vi "Create_setup_string.vi"() -> (0 "Setup String":string)   [LabVIEW 2017]
uses:
  Globals/Meas_global.vi
  Globals/Trav_pos_global.vi
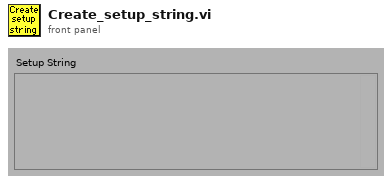
[diagram p1: front panel]
types:
  T1 = typedef "Analysis_info_cluster.ctl" = cluster{"Colour":u32, "Inst type":T2, "Inst name":string, "Symbol":string, "Code name":string, "Extra Info":string, "Inst Array":T3, "Extra Titles":string[], "Extra Values":string[], "U":dbl, "u^2":dbl, "u^3":dbl, "u^4":dbl, "Skew_u":dbl, "Kurt_u":dbl, "Sd Error in Mean":dbl, "% u'/U":dbl, "X":dbl, "Y":dbl, "Z":dbl, "Timescale integral Estimate":dbl, "Sd Error in Variance":dbl, "Calib File":path, "Calib Constants":dbl[], "Output Position":bool, "Full Stats":bool, "Av Sampling Rate":dbl, "Av No of Samples":dbl, "Total Meas Time (s)":dbl, "ADAM Ch Name":string, "Max value":dbl, "Min value":dbl, "Req Sample Rate Hz":dbl, "Sync Delay Time (s)":dbl, "Ch No":i16, "Device ID":string, "Use Latest Calib":bool}
  T2 = typedef "Inst_type.ctl" = enum16{"Propeller anemometer", "Raw voltage", "Pressure Transducer", "Pitot-static tube", "Preston tube", "Hot wire", "Cross wire 1", "Cross wire 2", "Generic Linear", "Generic Polynomial", "Generic BackPoly", "Fast FID", "Thermocouple", "Cold wire", "Pulsed Wire", "LDA Vel", "LDA Tran time", "LDA Arr time", "Microphone"}
  T3 = typedef "Instrument_Array.ctl" = enum16{"PWA", "LDA", "Analogue"}
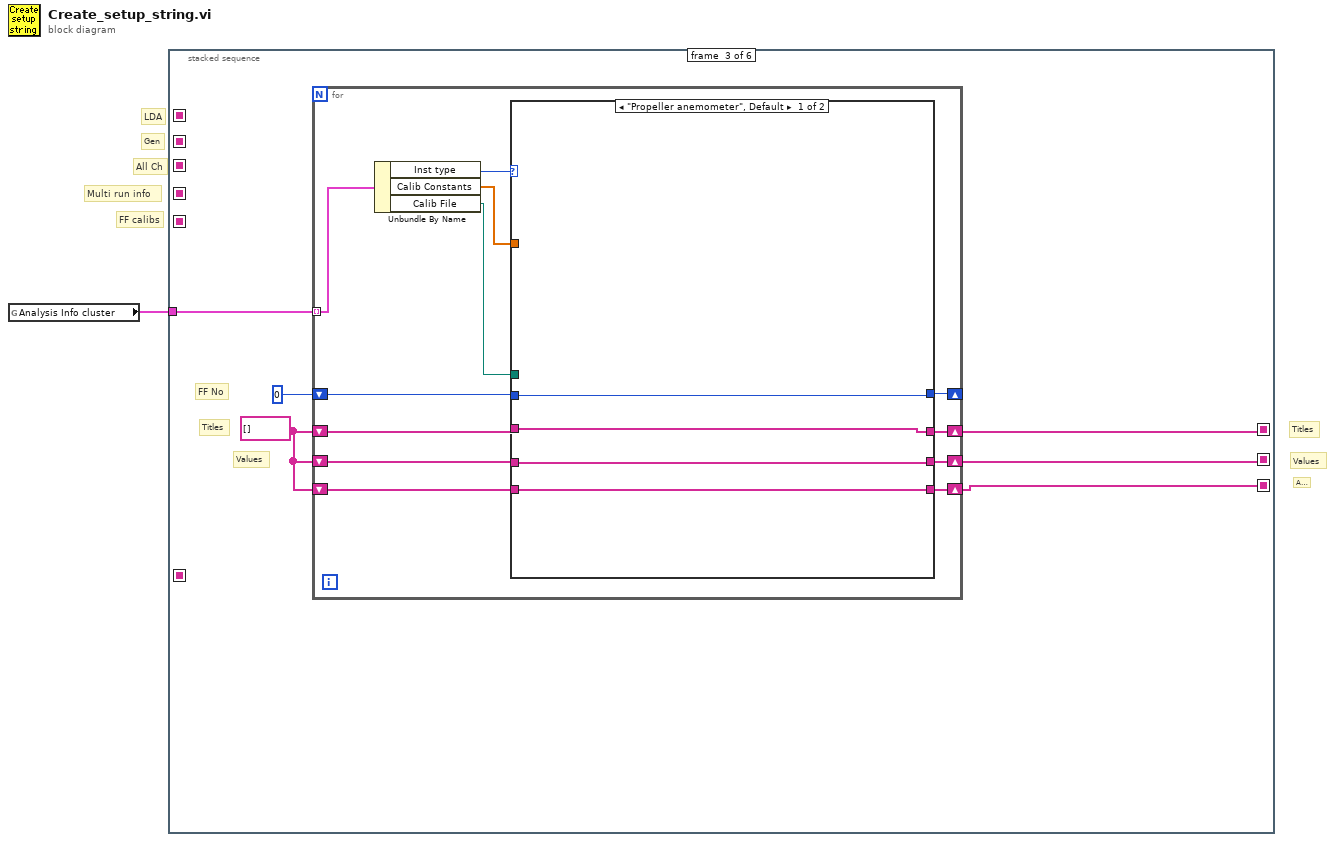
[diagram p0: block diagram]
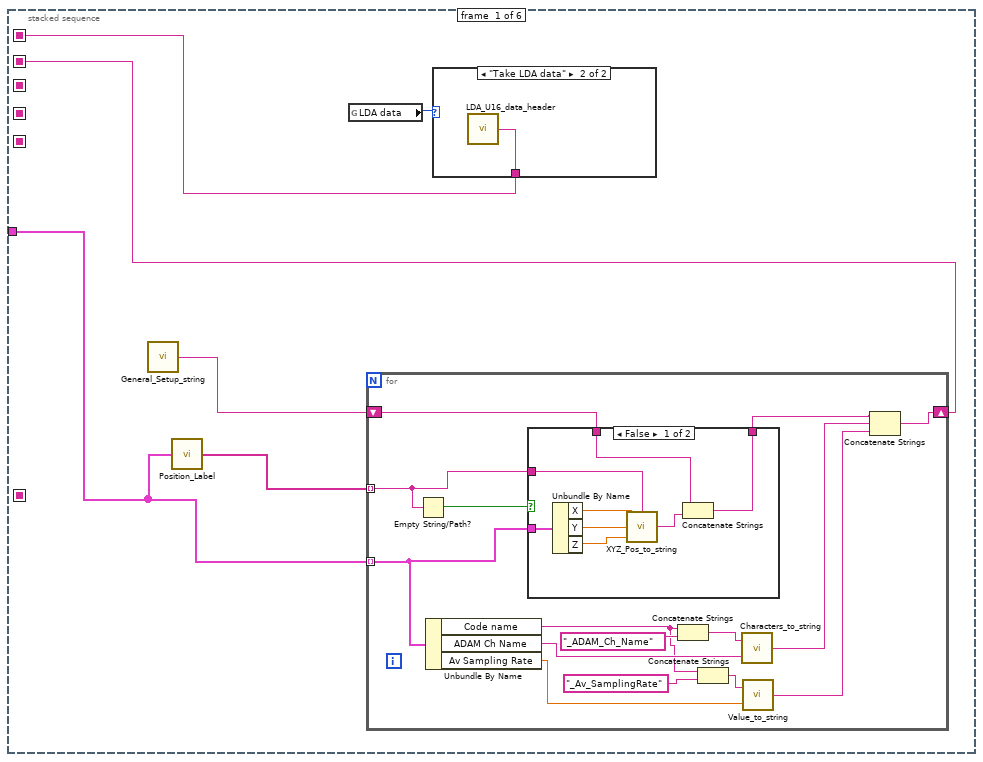
[diagram p2: hidden frame]
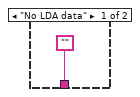
[diagram p4: hidden frame]
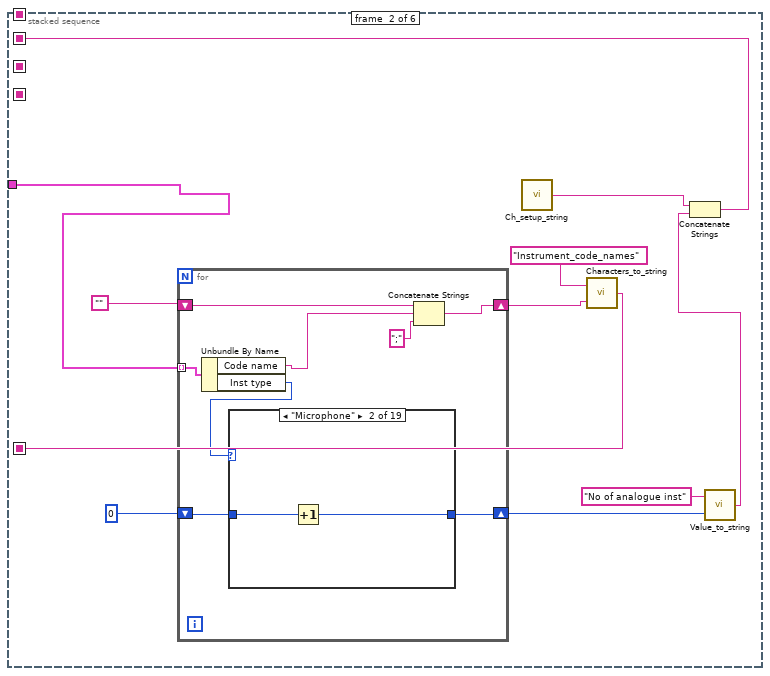
[diagram p5: hidden frame]
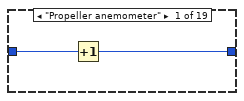
[diagram p6: hidden frame]
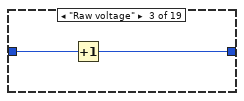
[diagram p7: hidden frame]
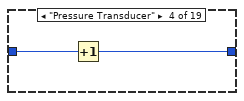
[diagram p8: hidden frame]
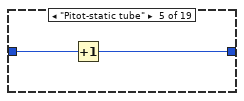
[diagram p9: hidden frame]
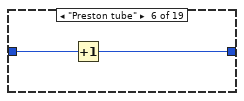
[diagram p10: hidden frame]
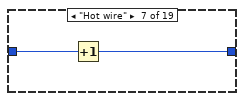
[diagram p11: hidden frame]
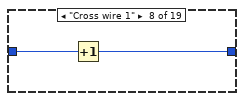
[diagram p12: hidden frame]
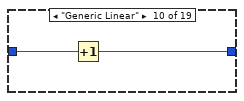
[diagram p14: hidden frame]
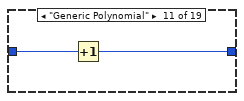
[diagram p15: hidden frame]
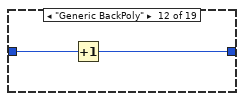
[diagram p16: hidden frame]
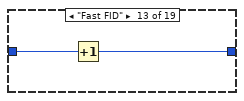
[diagram p17: hidden frame]
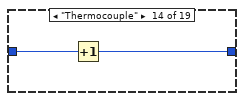
[diagram p18: hidden frame]
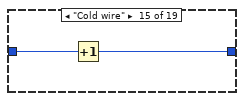
[diagram p19: hidden frame]
diagram:
  # "Multi run info"
  # "After"
  # "Values"
  # "Titles"
  # "FF calibs"
  # "LDA"
  # "Gen"
  # "All Ch"
  n1 = global read "Meas_global.vi" "Analysis Info cluster"() -> (w1:T1[])
  n2 = stacked-sequence {
    seq-local: [w7 _ _ _ _ _] -> [_ _ _ _ _ w221]
    seq-local: [w3 _ _ _ _ _] -> [_ _ _ _ _ w220]
    seq-local: [_ w35 _ _ _ _] -> [_ _ _ _ _ w219]
    seq-local: [_ _ _ _ w167 _] -> [_ _ _ _ _ w194]
    seq-local: [_ _ w89 _ _ _] -> [_ _ _ _ w168 _]
    seq-local: [_ _ w90 _ _ _] -> [_ _ _ _ w165 _]
    seq-local: [_ _ w87 _ _ _] -> [_ _ _ _ w163 _]
    seq-local: [_ w41 _ _ _ _] -> [_ _ _ _ _ w200]
    seq-local: [_ _ _ w155 _ _] -> [_ _ _ _ _ w193]
    tunnel: w1 -> [w2 w34 w86 _ _ _]
    frame #0 {
      n3 = call "General_Setup_string.vi"() -> ("Output string"=w4:string)  [unwired: 1 out]
      n4 = call "Position_Label.vi"("Analysis Info cluster"=w2) -> ("Position Label"=w5:string[])
      n5 = global read "Meas_global.vi" "LDA data"() -> (w6:enum16{"No LDA data", "Take LDA data"})
      n6 = for {
        shift-right: [w18] -> w3
        shift-left: w4 -> [w22]
        tunnel: w2 -> [w17] mode=indexing
        tunnel: w5 -> [w21] mode=indexing
        n7 = Empty String/Path?(string/path=w21) -> (empty?=w20:bool)
        n8 = Unbundle By Name(w17) -> ("Code name"=w11:string, "ADAM Ch Name"=w14:string, "Av Sampling Rate"=w12:dbl)
        n9 = case shown="False" w20 {
          tunnel: w22 -> [w30 w31]
          tunnel: [w29 w31] -> w19
          tunnel: w17 -> [w28 _]
          tunnel: w21 -> [w23 _]
          frame False {
            n10 = Unbundle By Name(w28) -> ("X"=w25:dbl, "Y"=w26:dbl, "Z"=w27:dbl)
            n11 = call "XYZ_Pos_to_string.vi"("Position label"=w23, "Z"=w27, "Y"=w26, "X"=w25) -> ("Output string"=w24:string)
            n12 = Concatenate Strings(w30, w24) -> (w29:string)
          }
          frame True {
          }
        }
        n13 = Concatenate Strings(w11, "_ADAM_Ch_Name" ("string")) -> (w15:string)
        n14 = Concatenate Strings(w11, "_Av_SamplingRate" ("string")) -> (w9:string)
        n15 = call "Characters_to_string.vi"("Characters to write"=w14, "Label for characters"=w15) -> ("Output string"=w13:string)
        n16 = call "Value_to_string.vi"("Value"=w12, "Label for value"=w9) -> ("Output string"=w8:string)  [unwired: 1 in]
        n17 = Concatenate Strings(w19, w13, w8) -> (w18:string)
      }
      n18 = case shown="\"Take LDA data\"" w6 {
        tunnel: ["" w33] -> w7
        frame "No LDA data" {
        }
        frame "Take LDA data" {
          n19 = call "LDA_U16_data_header.vi"() -> ("Output string"=w33:string)  [unwired: 1 out]
        }
      }
    }
    frame #1 {
      n20 = for {
        tunnel: w34 -> [w52] mode=indexing
        shift-right: [w48] -> w43
        shift-left: "" -> [w51]
        shift-right: [w45] -> w38
        shift-left: 0 -> [w46]
        n21 = Unbundle By Name(w52) -> ("Code name"=w50:string, "Inst type"=w47:T2)
        n22 = case shown="\"Microphone\"" w47 {
          tunnel: w46 -> [w54 w56 w58 w60 w62 w64 w66 w68 w69 w71 w73 w75 w77 w79 w81 w82 w83 w84 w85]
          tunnel: [w53 w55 w57 w59 w61 w63 w65 w67 w69 w70 w72 w74 w76 w78 w80 w82 w83 w84 w85] -> w45
          frame "Propeller anemometer" {
            n23 = Increment(x=w54) -> (x+1=w53:i32)
          }
          frame "Microphone" {
            n24 = Increment(x=w56) -> (x+1=w55:i32)
          }
          frame "Raw voltage" {
            n25 = Increment(x=w58) -> (x+1=w57:i32)
          }
          frame "Pressure Transducer" {
            n26 = Increment(x=w60) -> (x+1=w59:i32)
          }
          frame "Pitot-static tube" {
            n27 = Increment(x=w62) -> (x+1=w61:i32)
          }
          frame "Preston tube" {
            n28 = Increment(x=w64) -> (x+1=w63:i32)
          }
          frame "Hot wire" {
            n29 = Increment(x=w66) -> (x+1=w65:i32)
          }
          frame "Cross wire 1" {
            n30 = Increment(x=w68) -> (x+1=w67:i32)
          }
          frame "Cross wire 2" {
          }
          frame "Generic Linear" {
            n31 = Increment(x=w71) -> (x+1=w70:i32)
          }
          frame "Generic Polynomial" {
            n32 = Increment(x=w73) -> (x+1=w72:i32)
          }
          frame "Generic BackPoly" {
            n33 = Increment(x=w75) -> (x+1=w74:i32)
          }
          frame "Fast FID" {
            n34 = Increment(x=w77) -> (x+1=w76:i32)
          }
          frame "Thermocouple" {
            n35 = Increment(x=w79) -> (x+1=w78:i32)
          }
          frame "Cold wire" {
            n36 = Increment(x=w81) -> (x+1=w80:i32)
          }
          frame "Pulsed Wire" {
          }
          frame "LDA Vel" {
          }
          frame "LDA Tran time" {
          }
          frame "LDA Arr time" {
          }
        }
        n37 = Concatenate Strings(w51, w50, ";" ("string")) -> (w48:string)
      }
      n38 = call "Ch_setup_string.vi"() -> ("Output string"=w37:string)  [unwired: 3 in, 3 out]
      n39 = call "Characters_to_string.vi"("Characters to write"=w43, "Label for characters"="Instrument_code_names") -> ("Output string"=w41:string)
      n40 = call "Value_to_string.vi"("Value"=w38, "Label for value"="No of analogue inst") -> ("Output string"=w36:string)  [unwired: 1 in]
      n41 = Concatenate Strings(w37, w36) -> (w35:string)
    }
    frame #2 {
      w88 = string[] []
      # "Values"
      # "Titles"
      # "FF No"
      n42 = for {
        shift-right: [w99] -> w89
        shift-left: w88 -> [w100]
        shift-right: [w101] -> _
        shift-left: 0 -> [w102]
        shift-right: [w97] -> w90
        shift-left: w88 -> [w98]
        shift-right: [w95] -> w87
        shift-left: w88 -> [w96]
        tunnel: w86 -> [w92] mode=indexing
        n43 = Unbundle By Name(w92) -> ("Inst type"=w103:T2, "Calib Constants"=w94:dbl[], "Calib File"=w93:path)
        n44 = case shown="\"Propeller anemometer\", Default" w103 {
          tunnel: w94 -> [_ w117]
          tunnel: w93 -> [_ w116]
          tunnel: w102 -> [w107 w115]
          tunnel: [w107 w114] -> w101
          tunnel: w100 -> [w106 w113]
          tunnel: [w106 w112] -> w99
          tunnel: w98 -> [w105 w111]
          tunnel: [w105 w110] -> w97
          tunnel: w96 -> [w104 w109]
          tunnel: [w104 w108] -> w95
          frame "Propeller anemometer", Default {
          }
          frame "Fast FID" {
            n45 = stacked-sequence {
              seq-local: [w118 _] -> [_ w140]
              tunnel: w117 -> [_ w153]
              tunnel: w116 -> [_ w154]
              tunnel: w115 -> [w133 _]
              tunnel: [w118 _] -> w114
              tunnel: w113 -> [w129 _]
              tunnel: [w128 _] -> w112
              tunnel: w111 -> [_ w148]
              tunnel: [_ w147] -> w110
              tunnel: w109 -> [_ w145]
              tunnel: [_ w144] -> w108
              frame #0 {
                # "Titles"
                n46 = Increment(x=w133) -> (x+1=w118:i32)
                n47 = Number To Decimal String(number=w118) -> (decimal integer string=w119:string)  [unwired: 1 out]
                n48 = Build Array("Calib Filename", "Coeff A", "Coeff B", "Coeff C", "Bkgnd", "Bkgnd Variance", "Bkgnd Volts", "Bkgnd Time") -> (w130:string[])
                n49 = for {
                  tunnel: "FF:" -> [w138]
                  tunnel: w119 -> [w137]
                  tunnel: w130 -> [w135] mode=indexing
                  tunnel: [w134] -> w122 mode=indexing
                  n50 = Concatenate Strings(w138, w137, ":" ("Substring"), w135) -> (w134:string)
                }
                n51 = Build Array (concatenate)(w129, w122) -> (w128:string[])
              }
              frame #1 {
                n52 = Array Subset(array=w153, length=7 ("Array Length")) -> (w151:dbl[])  [unwired: 1 in]
                n53 = Initialize Array("", 4 ("dimension size")) -> (w141:string[])
                n54 = call "Bkgnd_place_names.vi"("Numeric"=w140) -> ("Array"=w139:string[])
                n55 = Path To String(path=w154) -> (string=w146:string)
                n56 = Number To Fractional String(number=w151, precision (6)=i16 10) -> (F-format string=w149:string[])  [unwired: 2 out]
                n57 = Build Array (concatenate)(w148, w146, w149) -> (w147:string[])
                n58 = Build Array (concatenate)(w145, w141, w139) -> (w144:string[])
              }
            }
          }
        }
      }
    }
    frame #3 {
      n59 = global read "Trav_pos_global.vi" "Current Image Filename"() -> (w160:path)
      n60 = global read "Meas_global.vi" "Extra command String"() -> (w162:string)
      n61 = call "Path_2_String.vi"("Real Path"=w160) -> ("Path String"=w159:string)
      n62 = call "Characters_to_string.vi"("Characters to write"=w162, "Label for characters"="Meas_Global.vi_Extra Command String") -> ("Output string"=w157:string)
      n63 = call "Characters_to_string.vi"("Characters to write"=w159, "Label for characters"="Trav_pos_global.vi_Current Image Filename") -> ("Output string"=w156:string)
      n64 = Concatenate Strings(w157, w156) -> (w155:string)
    }
    frame #4 {
      n65 = Array Size(array=w165) -> (size(s)=w166:i32)
      n66 = Not Equal To 0?(x=w166) -> (x != 0?=w164:bool)
      n67 = case shown="True" w164 {
        tunnel: w168 -> [_ w185]
        tunnel: w165 -> [_ w179]
        tunnel: ["" w173] -> w167
        tunnel: w163 -> [_ w171]
        frame False {
        }
        frame True {
          n68 = Build Array (concatenate)("FF:Calib:History" ("Input Element"), w185) -> (w176:string[])
          n69 = for {
            tunnel: w176 -> [w192] mode=indexing
            tunnel: [w191] -> w188 mode=indexing
            tunnel: [w190] -> w187 mode=indexing
            tunnel: [w189] -> w186 mode=indexing
            n70 = call "Split_Ch_name.vi"("Ch name"=w192) -> ("Top level"=w191:string, "Middle"=w190:string, "Low level"=w189:string)
          }
          n71 = Build Array (concatenate)("Calibration To be Used" ("Input Element"), w179) -> (w181:string[])
          n72 = call "Asterisk_header.vi"("Channel names"=w176) -> ("Header string"=w174:string)
          n73 = Build Array (concatenate)("Calibration After Meas" ("Input Element"), w171) -> (w170:string[])
          n74 = Build Array (concatenate)("Calibration Before Meas" ("Input Element"), w179) -> (w182:string[])
          n75 = Build Array(w188, w187, w186, w182, w170, w181) -> (w177:string[][])
          n76 = Array To Spreadsheet String(array=w177, 3:"%s" ("format string")) -> (spreadsheet string=w175:string)  [unwired: 1 out]
          n77 = Concatenate Strings(w174, w175) -> (w173:string)
        }
      }
    }
    frame #5 {
      w195 = "Initial Probe positions" ("File Label")
      n78 = global read "Meas_global.vi" "Pre Setup String"() -> (w199:string)
      n79 = Get Date/Time In Seconds() -> (seconds since 1Jan1904=w207:timestamp)
      n80 = To Double Precision Float(number=w207) -> (double precision float=w209:dbl)
      n81 = global read "Meas_global.vi" "New Setup String"() -> (w197:string)
      n82 = global read "Meas_global.vi" "Results file"() -> (w216:path)
      n83 = call "Get_string_subset.vi"("String to split"=w199, "File Label"=w195) -> ("Output string"=w198:string)  [unwired: 2 in, 1 out]
      n84 = Number To Fractional String(number=w209, precision (6)=i16 0) -> (F-format string=w206:string)  [unwired: 2 out]
      n85 = Path To String(path=w216) -> (string=w213:string)
      n86 = call "Characters_to_string.vi"("Characters to write"=w206, "Label for characters"="Measurement_End_Time_Seconds") -> ("Output string"=w204:string)
      n87 = call "Characters_to_string.vi"("Characters to write"="", "Label for characters"="Skip_Block_Numbers_(eg 1;2;5;12)" ("Variable name")) -> ("Output string"=w201:string)
      n88 = call "Add_label_to_string.vi"("String to write"=w198, "File Label"=w195) -> ("Output string"=w196:string)
      n89 = call "Characters_to_string.vi"("Characters to write"=w213, "Label for characters"="Results filename") -> ("Output string"=w217:string)
      n90 = Concatenate Strings(w197, w196, w204, w217, w221, w220, w219, w193, w194, w201, w200) -> (w211:string)
      n91 = call "Add_label_to_string.vi"("String to write"=w211, "File Label"="Raw data header") -> ("Output string"=→"Setup String":string)
      n92 = Concatenate Strings("\r\n", w211) -> (w212:string)
      n93 = global write "Meas_global.vi" "New Setup String"(w212) -> ()
    }
  }
